vi "Withdraw.vi"(8 "error in (no error)":errorcluster, 10 "Amount":dbl, 11 "ASavings in":refnum<class "ASavings.lvclass">) -> (0 "error out":errorcluster, 1 "Success?":bool, 2 "Balance":dbl, 3 "ASavings out":refnum<class "ASavings.lvclass">)   [LabVIEW 2020, in "ASavings.lvclass"]
uses:
  ASavings.lvclass
  ASavings.lvclass/ASavings.ctl
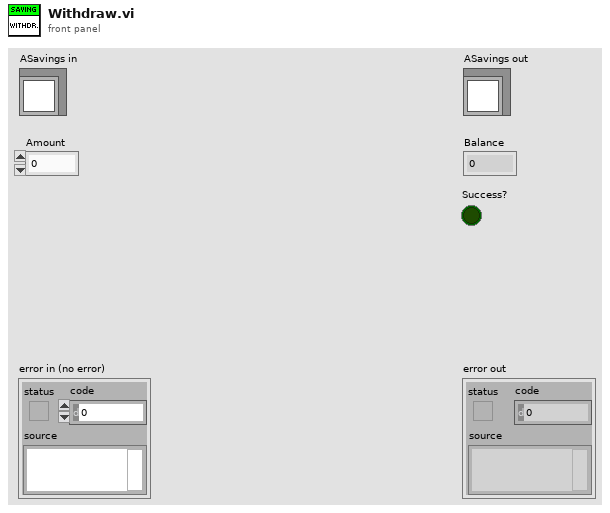
[diagram p1: front panel]
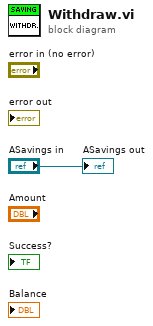
[diagram p0: block diagram]
diagram:
  "ASavings out" <- "ASavings in"
